vi "XIPIN_3GPPLTE_Turbo_Encoder_4_0.vi"   [LabVIEW 2017]
doc: "The Turbo Encoder IP from Xilinx is a high-speed, compact Turbo Encoder which meets the 3GPP LTE specification.\n------------------------------------\n<b>Need License</b> : Yes"
uses:
  <vilib>/rvi/XilinxIP/XIPIN_XNode/niFpgaXIPIN.xnode
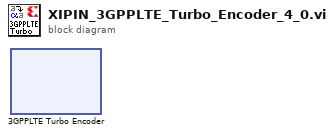
[diagram p0: block diagram]
diagram:
  n1 = xnode ("3GPPLTE Turbo Encoder")() -> ()
